vi "Write File Path.vi"(8 "error in (no error)":errorcluster, 10 "File Path":path, 11 "Parameter Generic File in":refnum<class "Parameter Generic File.lvclass">) -> (0 "error out":errorcluster, 3 "Parameter Generic File out":refnum<class "Parameter Generic File.lvclass">)   [LabVIEW 2016, in "CD Parameter Manager API.lvlib" / "Parameter Generic File.lvclass"]
uses:
  Parameter Generic File.lvclass
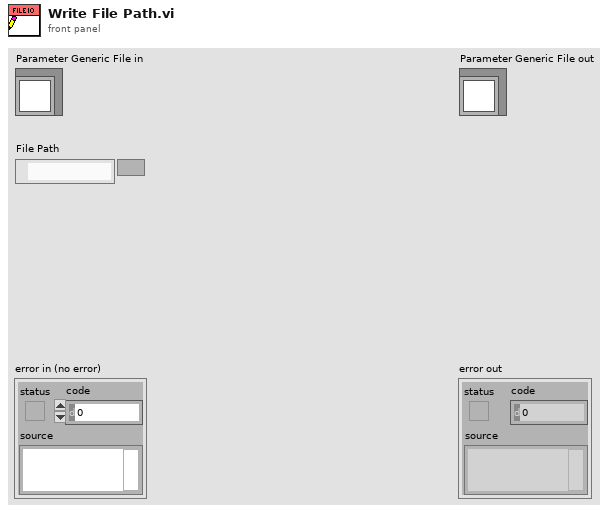
[diagram p1: front panel]
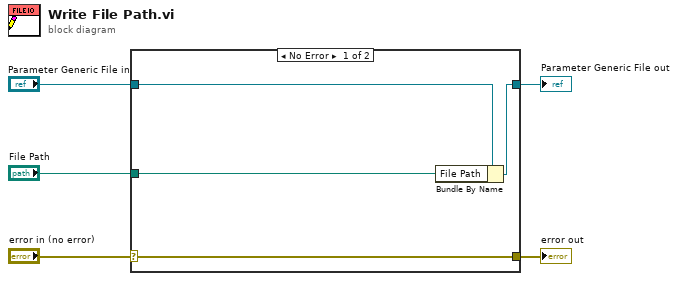
[diagram p0: block diagram]
diagram:
  n1 = case shown="No Error" "error in (no error)" {
    selector: "error in (no error)" -> [w9 w10]
    tunnel: [w9 w10] -> w4
    tunnel: [w7 w11] -> w2
    tunnel: "Parameter Generic File in" -> [w8 w11]
    tunnel: "File Path" -> [w6 _]
    frame No Error {
      n2 = Bundle By Name(cluster=w8, "File Path"=w6) -> (w7:refnum<class "Parameter Generic File.lvclass">)
    }
    frame Error {
    }
  }
  "error out" <- w4
  "Parameter Generic File out" <- w2
